vi "PalmSense Configure LSV.vi"(8 "error in (no error)":errorcluster, 10 "Message Data":variant, 11 "Data Cluster in":T1) -> (0 "error out":errorcluster, 3 "Data Cluster out":T1)   [LabVIEW 2020, in "PalmSens.lvlib"]
uses:
  PalmSens.lvlib
  PalmSense Hardware Configuration.ctl
  <instrlib>/PalmSens SDK for LabVIEW 5.10/PalmSens/PalmSens.lvclass
  support/Message Queue/Message Cluster.ctl
  support/HW Message Cluster.ctl
  C:/Program Files (x86)/National Instruments/LabVIEW 2020/instr.lib/PalmSens SDK for LabVIEW 5.10/PalmSens/Libraries/PalmSens.Core.dll
  support/Message Queue/Message Queue.lvlib
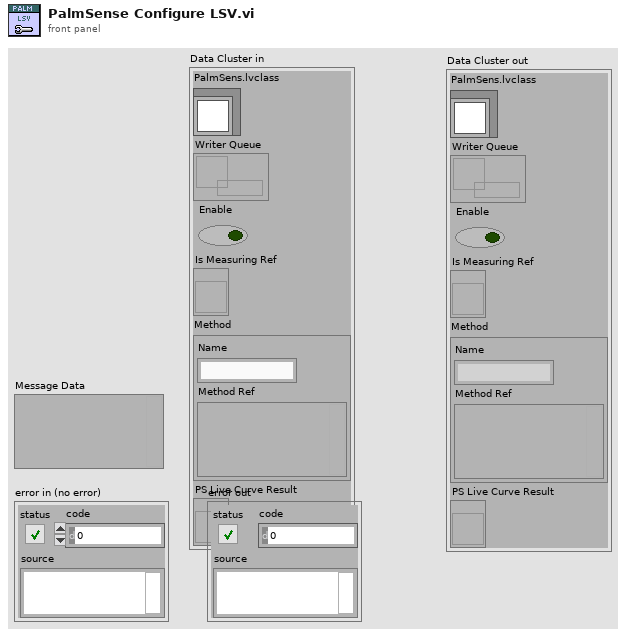
[diagram p1: front panel]
types:
  T1 = typedef "PalmSens.lvlib/PalmSense Hardware Configuration.ctl" = cluster{"PalmSens.lvclass":refnum<class "PalmSens.lvclass">, "Writer Queue":refnum<queue>, "Enable":bool, "Is Measuring Ref":refnum<vi>, "Method":cluster{"Name":string, "Method Ref":variant}, "PS Live Curve Result":refnum<vi>}
  T2 = cluster{"BeginPotential":sgl, "EndPotential":sgl, "StepPotential":sgl, "Scanrate":sgl}
  T3 = typedef "Message Queue.lvlib/HW Message Cluster.ctl" = cluster{"Writer Queue":refnum<queue>, "Writer Data":T4}
  T4 = typedef "Message Queue.lvlib/Message Cluster.ctl" = cluster{"Message":string, "Message Data":variant}
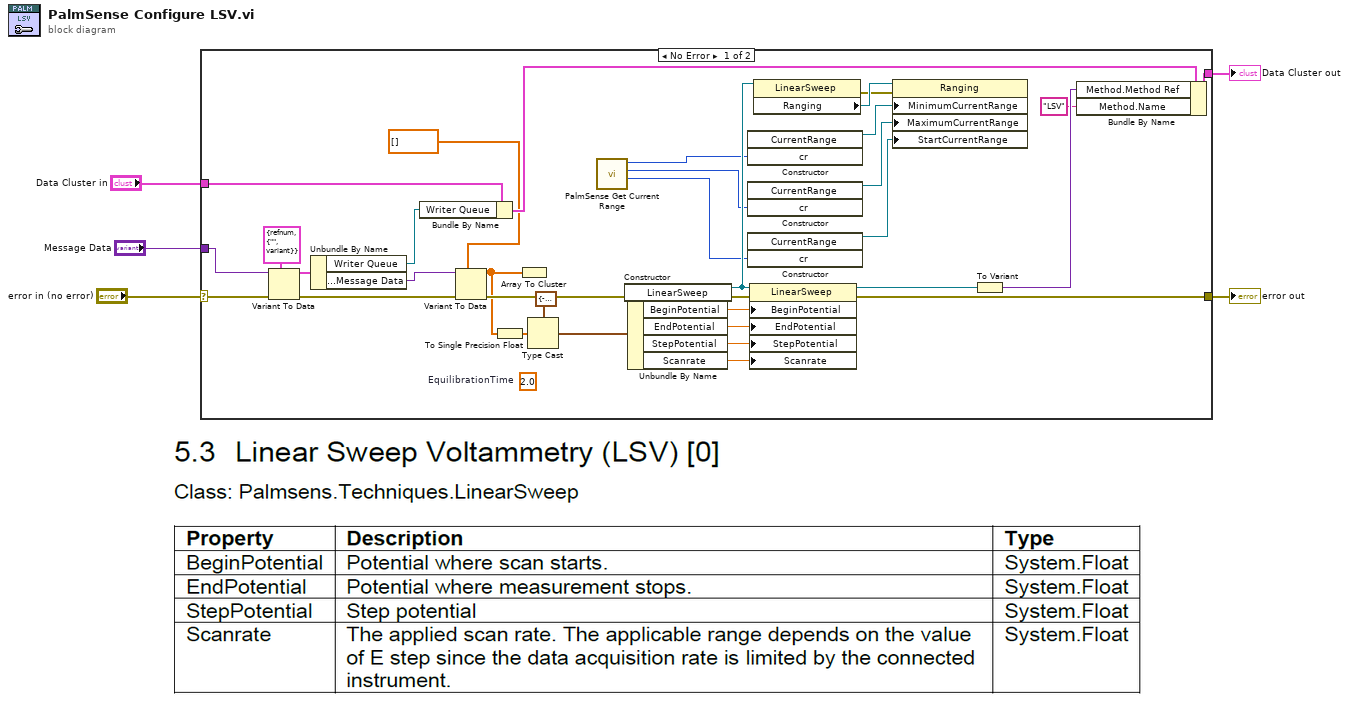
[diagram p0: block diagram]
diagram:
  n1 = case shown="No Error" "error in (no error)" {
    selector: "error in (no error)" -> [w36 w40]
    tunnel: "Message Data" -> [w34 _]
    tunnel: [w17 w41] -> w4
    tunnel: "Data Cluster in" -> [w38 w41]
    tunnel: [w22 w40] -> w2
    frame No Error {
      (unwired) sgl 2.0  # EquilibrationTime
      n2 = Variant To Data(error in=w36, type=T3 {"Writer Queue"=refnum, "Writer Data"={"Message"="", "Message Data"=variant}}, Variant=w34) -> (data=w37:T3, error out=w35:errorcluster)
      n3 = Unbundle By Name(w37) -> ("Writer Queue"=w32:refnum<queue>, "Writer Data.Message Data"=w33:variant)
      n4 = Bundle By Name(cluster=w38, "Writer Queue"=w32) -> (w39:T1)
      n5 = Variant To Data(error in=w35, type=dbl[] [] ("LSV Scan"), Variant=w33) -> (data=w12:dbl[], error out=w30:errorcluster)
      n6 = To Single Precision Float(number=w12) -> (single precision float=w6:sgl[])
      n7 = Array To Cluster(array=w12) -> ()  [unwired: 1 out]
      n8 = Type Cast(type=T2 {"BeginPotential"=-1.0, "EndPotential"=1.0, "StepPotential"=0.01, "Scanrate"=0.5}, x=w6) -> (*(type *) &x=w10:T2)
      n9 = call "PalmSense Get Current Range.vi"() -> ("Start Current Range"=w9:i32, "Max Current Range"=w8:i32, "Min Current Range"=w7:i32)  [unwired: 9 in]
      n10 = constructor class="LinearSweep"(error in=w30) -> (reference out=w24:refnum<k24>, error out=w21:errorcluster)  [unwired: 2 in, 1 out]
      n11 = Unbundle By Name(w10) -> ("BeginPotential"=w23:sgl, "EndPotential"=w20:sgl, "StepPotential"=w19:sgl, "Scanrate"=w18:sgl)
      n12 = constructor class="CurrentRange"("cr"=w7) -> (reference out=w27:refnum<k24>)  [unwired: 3 in, 3 out]
      n13 = constructor class="CurrentRange"("cr"=w8) -> (reference out=w28:refnum<k24>)  [unwired: 3 in, 3 out]
      n14 = constructor class="CurrentRange"("cr"=w9) -> (reference out=w29:refnum<k24>)  [unwired: 3 in, 3 out]
      n15 = property class="LinearSweep"(reference=w24, error in=w21, "BeginPotential"=w23, "EndPotential"=w20, "StepPotential"=w19, "Scanrate"=w18) -> (reference out=w16:refnum<k24>, error out=w22:errorcluster)
      n16 = property class="LinearSweep"(reference=w24) -> (error out=w25:errorcluster, "Ranging"=w26:refnum<k24>)  [unwired: 1 in, 1 out]
      n17 = property class="Ranging"(reference=w26, error in=w25, "MinimumCurrentRange"=w27, "MaximumCurrentRange"=w28, "StartCurrentRange"=w29) -> ()  [unwired: 2 out]
      n18 = To Variant(anything=w16) -> (Variant=w15:variant)
      n19 = Bundle By Name(cluster=w39, "Method.Method Ref"=w15, "Method.Name"="LSV") -> (w17:T1)
    }
    frame Error {
    }
  }
  "Data Cluster out" <- w4
  "error out" <- w2
